vi "MotorFunc.vi"(6 "停止":bool, 8 "error in (no error)":errorcluster, 11 "把当前坐标系下期望小\n车在X、Y、θ的速度作\n为逆运算的输入":dbl[](array[numeric])=[0.0, 0.0, 0.0]) -> (0 "error out":errorcluster, 3 "真实坐标系下的X、Y、θ的速度":dbl[](array[numeric]))   [LabVIEW 2017]
uses:
  <vilib>/robotics/Steering/Differential Steering Frame/NI_Robotics_Differential Steering Frame.lvclass
  E:/National Instruments/LabVIEW 2017/vi.lib/robotics/Steering/Steering Frame/NI_Robotics_Steering Frame.lvclass
  <vilib>/robotics/Steering/Steering Frame/Apply Steering Frame Velocity to Motors.vi
  <vilib>/robotics/Steering/Steering Frame/Get Steering Frame Velocity from Motors.vi
  <vilib>/robotics/Steering/Steering Frame/NI_Robotics_Steering Frame.lvclass
  E:/National Instruments/LabVIEW 2017/vi.lib/robotics/Steering/Special Steering Frame/NI_Robotics_Special Steering Frame.lvclass
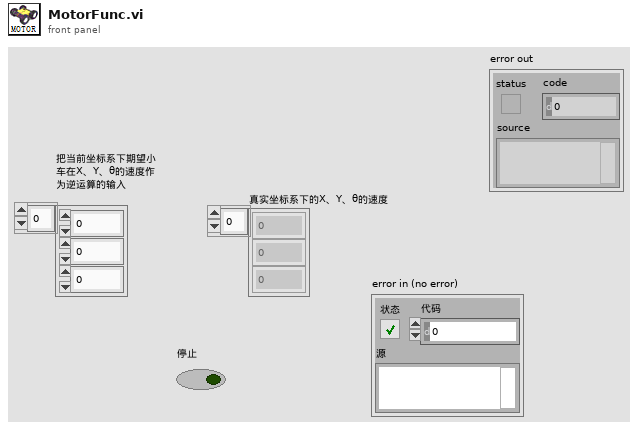
[diagram p1: front panel]
types:
  T1 = typedef "NI_Robotics_Steering Class Types.lvlib/Differential Steering Frame.ctl" = refnum<class "NI_Robotics_Differential Steering Frame.lvclass">
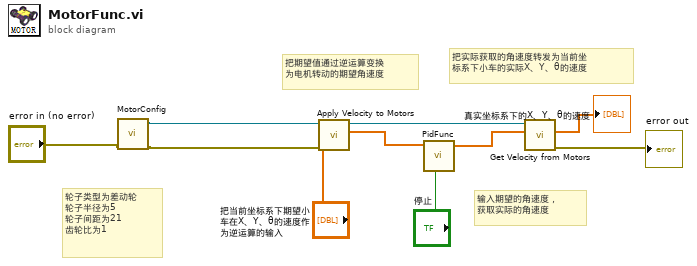
[diagram p0: block diagram]
diagram:
  # "把实际获取的角速度转发为当前坐\n标系下小车的实际X、Y、θ的速度"
  # "输入期望的角速度，\n获取实际的角速度"
  # "把期望值通过逆运算变换\n为电机转动的期望角速度"
  # "轮子类型为差动轮\n轮子半径为5\n轮子间距为21\n齿轮比为1"
  n1 = call "MotorConfig.vi"("error in (no error)"="error in (no error)") -> ("error out"=w1:errorcluster, "differential steering frame out"=w2:T1)  [unwired: 9 in]
  n2 = call-poly <vilib>:"Apply Velocity to Motors.vi"("error in (no error)"=w1, "steering frame velocity"="把当前坐标系下期望小\n车在X、Y、θ的速度作\n为逆运算的输入", "steering frame in"=w2) -> ("ccw motor velocity setpoints"=w9:dbl[], "steering frame out"=w7:T1)  [unwired: 4 in, 3 out]
  n3 = call "PidFunc.vi"("刹车"="停止", "运用学解算后得\n到的两个电机\n的期望角速度"=w9) -> ("得到电机转动的角速度"=w10:dbl[])  [unwired: 9 in]
  n4 = call-poly <vilib>:"Get Velocity from Motors.vi"("ccw motor velocity states"=w10, "steering frame in"=w7) -> ("error out"=→"error out":errorcluster, "estimated steering frame velocity"=→"真实坐标系下的X、Y、θ的速度":dbl[])  [unwired: 7 in, 1 out]
